vi "低层函数-sequrnce.vi"() -> ()   [LabVIEW 2018]
uses:
  <vilib>/userdefined/High Color/IMAQdx.ctl
  <vilib>/vision/Image Controls.llb/IMAQ Image.ctl
  <vilib>/vision/driver/IMAQdx.llb/IMAQdx Acquisition Mode.ctl
  <vilib>/vision/driver/IMAQdx.llb/IMAQdx Buffer Number Mode.ctl
  <vilib>/vision/driver/NI_Vision_Acquisition_Software.lvlib
panel:
  out "数组":T1[](array[typedef])
  in  "Number of Buffers":u32=1
  in  "数值":i32
  out "error out":errorcluster
  in  "error in":errorcluster
  in  "Session In":T2
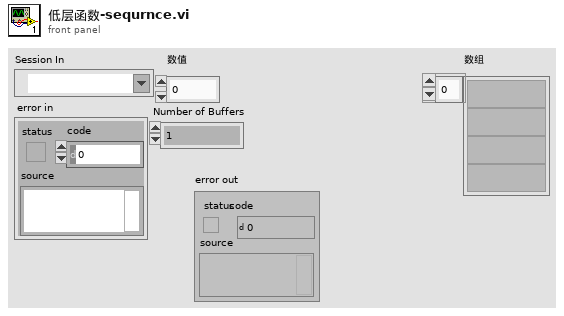
[diagram p1: front panel]
types:
  T1 = typedef "IMAQ Image.ctl" = refnum<image>
  T2 = typedef "IMAQdx.ctl" = refnum<k21>
  T3 = typedef "NI_Vision_Acquisition_Software.lvlib/IMAQdx Acquisition Mode.ctl" = enum32{"One Shot", "Continuous"}
  T4 = typedef "NI_Vision_Acquisition_Software.lvlib/IMAQdx Buffer Number Mode.ctl" = enum32{"Next", "Last", "Buffer Number", "Every", "Last New"}
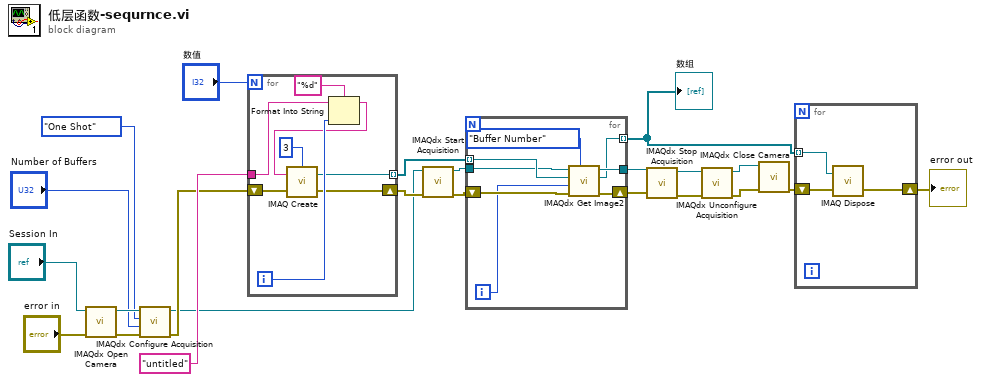
[diagram p0: block diagram]
diagram:
  n1 = call <vilib>:"IMAQdx Open Camera.vi"("error in"="error in", "Session In"="Session In") -> ("error out"=w16:errorcluster, "Session Out"=w17:T2)  [unwired: 8 in]
  n2 = call <vilib>:"IMAQdx Configure Acquisition.vi"("error in"=w16, "Number of Buffers"="Number of Buffers", "Continuous?"=IMAQdx_Acquisition_Mode."One Shot", "Session In"=w17) -> ("error out"=w15:errorcluster, "Session Out"=w14:T2)  [unwired: 6 in]
  n3 = for {
    N: "数值" -> [_]
    tunnel: "untitled" ("Image Name") -> [w29]
    shift-right: [w25] -> w18
    shift-left: w15 -> [w31]
    tunnel: [w24] -> w13 mode=indexing
    i -> [w28]
    n4 = Format Into String(format string="%d" ("格式字符串"), initial string=w29, w28) -> (resulting string=w26:string)  [unwired: 1 in, 1 out]
    n5 = call "IMAQ Create"("Border Size"=3, "Image Name"=w26, "error in (no error)"=w31) -> ("New Image"=w24:T1, "error out"=w25:errorcluster)  [unwired: 2 in]
  }
  n6 = call <vilib>:"IMAQdx Start Acquisition.vi"("error in"=w18, "Session In"=w14) -> ("error out"=w11:errorcluster, "Session Out"=w12:T2)  [unwired: 8 in]
  n7 = for {
    tunnel: w13 -> [w39] mode=indexing
    tunnel: w12 -> [w38]
    shift-right: [w36] -> w9
    shift-left: w11 -> [w37]
    tunnel: [w33] -> w10
    tunnel: [w32] -> w1 mode=indexing
    i -> [w34]
    n8 = call <vilib>:"IMAQdx Get Image2.vi"("Buffer Number Mode (Next)"=IMAQdx_Buffer_Number_Mode."Buffer Number", "error in"=w37, "Buffer Number In"=w34, "Image In"=w39, "Session In"=w38) -> ("error out"=w36:errorcluster, "Image Out"=w32:T1, "Session Out"=w33:T2)  [unwired: 3 in, 1 out]
  }
  "数组" <- w1
  n9 = call <vilib>:"IMAQdx Stop Acquisition.vi"("error in"=w9, "Session In"=w10) -> ("error out"=w8:errorcluster, "Session Out"=w6:T2)  [unwired: 8 in]
  n10 = call <vilib>:"IMAQdx Unconfigure Acquisition.vi"("error in"=w8, "Session In"=w6) -> ("error out"=w7:errorcluster, "Session Out"=w5:T2)  [unwired: 8 in]
  n11 = call <vilib>:"IMAQdx Close Camera.vi"("error in"=w7, "Session In"=w5) -> ("error out"=w20:errorcluster)  [unwired: 9 in]
  n12 = for {
    shift-right: [w41] -> w4
    shift-left: w20 -> [w42]
    tunnel: w1 -> [w40] mode=indexing
    n13 = call "IMAQ Dispose"("Image"=w40, "error in (no error)"=w42) -> ("error out"=w41:errorcluster)  [unwired: 4 in]
  }
  "error out" <- w4
